vi "AV Write Single.vi"(8 "error in":errorcluster, 9 "Channel Index":i32=1, 10 "Current AV":dbl, 11 "Current Actual Value in":refnum<class "Current Actual Value.lvclass">) -> (0 "error out":errorcluster, 3 "Current Actual Value out":refnum<class "Current Actual Value.lvclass">)   [LabVIEW 2023, in "Current Actual Value.lvclass"]
uses:
  Current Actual Value.lvclass
  Parents/Actual Value/Actual Value.lvclass
  Current Actual Value.lvclass/Current Actual Value.ctl
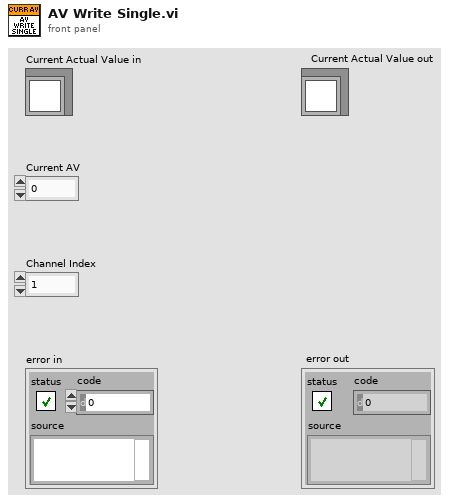
[diagram p1: front panel]
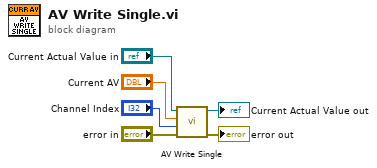
[diagram p0: block diagram]
diagram:
  n1 = call-parent "AV Write Single.vi"("error in"="error in", "Channel Index"="Channel Index", "Actual Value"="Current AV", "Actual Value in"="Current Actual Value in") -> ("error out"=→"error out":errorcluster, "Actual Value out"=→"Current Actual Value out":refnum<class "Current Actual Value.lvclass">)  [unwired: 6 in]
